vi "Convert Sense Mode.vi"(0 "Sense":T1 items=["Local", "Remote"]) -> (4 "Measurement:Sense":i32)   [LabVIEW 2024, in "devicePowerSequencerCoreLogic.lvlib"]
uses:
  devicePowerSequencerCoreLogic.lvlib
  controls/Sense Mode.ctl
  Device Power Sequencer.lvlib
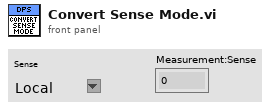
[diagram p1: front panel]
types:
  T1 = typedef "Device Power Sequencer.lvlib/Sense Mode.ctl" = i32
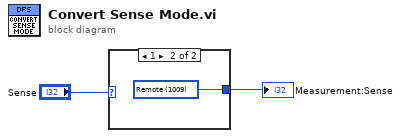
[diagram p0: block diagram]
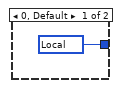
[diagram p2: hidden frame]
diagram:
  n1 = case shown="1" "Sense" {
    tunnel: [w3 w4] -> w1
    frame 0, Default {
      w3 = 1008 items=["Local"=1008, "Remote"=1009] ("Measurement:Sense")
    }
    frame 1 {
      w4 = 1009 items=["Local"=1008, "Remote"=1009] ("Measurement:Sense")
    }
  }
  "Measurement:Sense" <- w1
